vi "e.gate ReadeStateInfo.vi"(0 "Configuration  in":T1, 5 "error in (no error)":errorcluster) -> (14 "Configuration out":T1, 15 "data string":string, 16 "General States":string, 17 "Run States":string, 18 "Error States":string, 19 "error out":errorcluster)   [LabVIEW 2016]
uses:
  e.gate Configuration.ctl
  e.gate Channel Data.ctl
  e.gate Data Type.ctl
  e.gate Protocol Type.ctl
  e.gate Module  Data.ctl
  e.gateHSP_DLLhandle.ctl
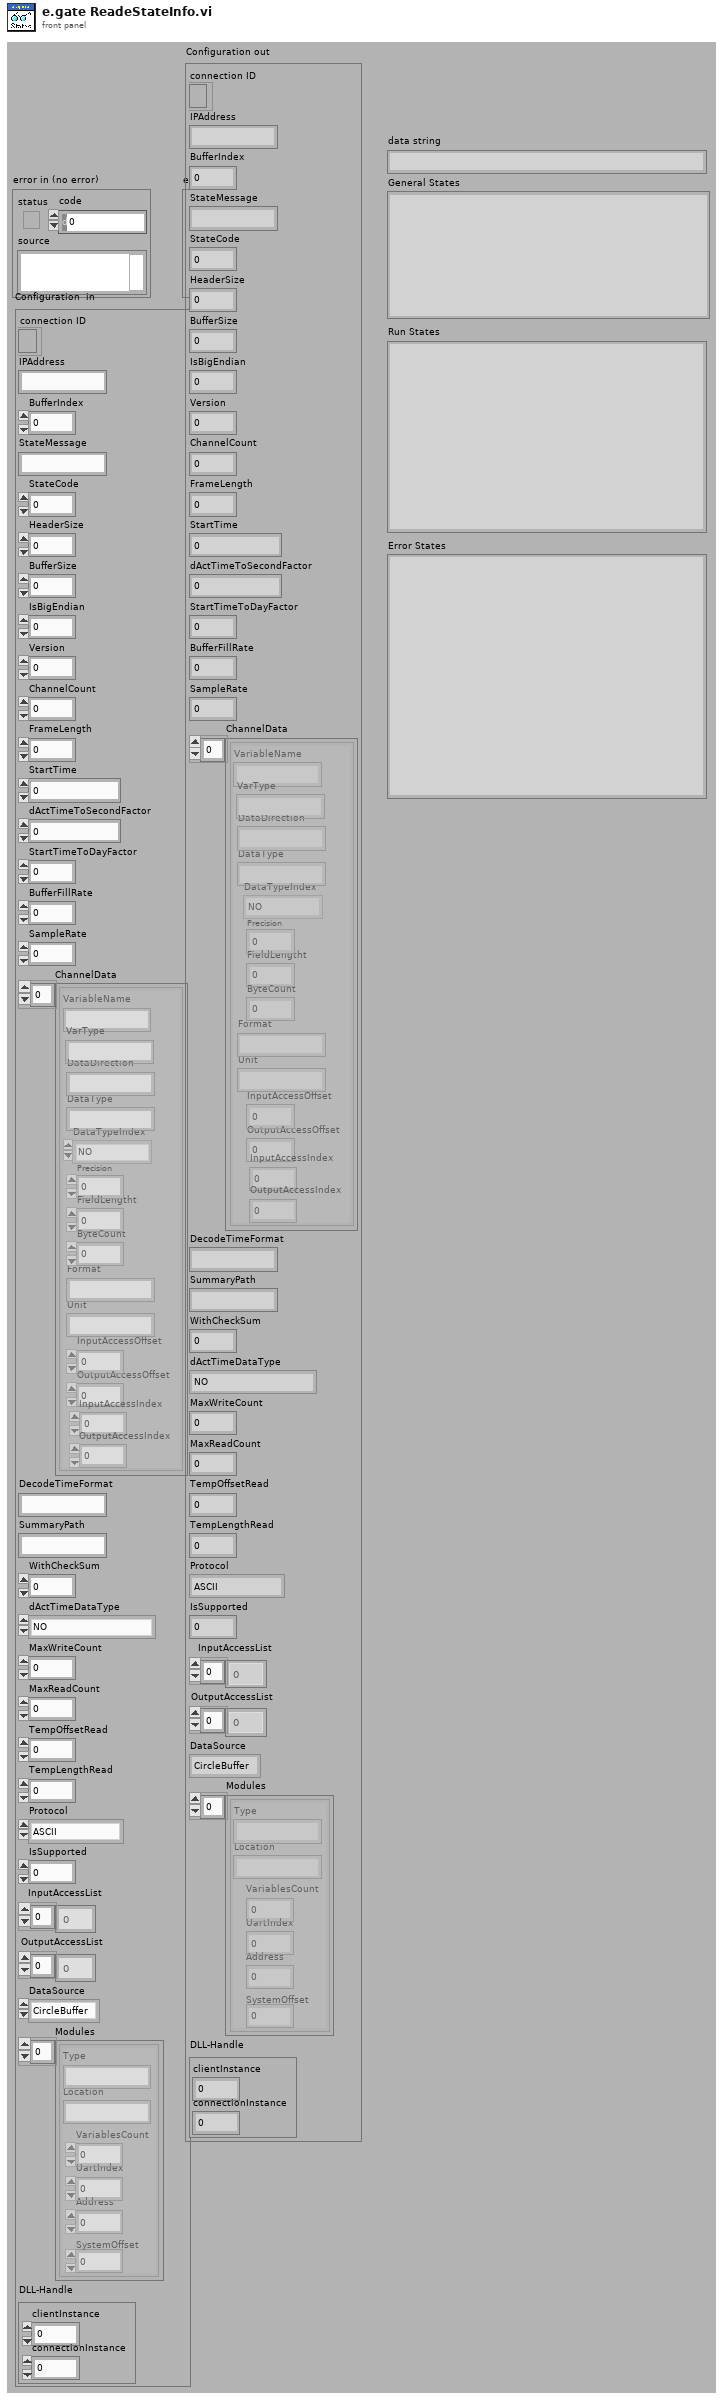
[diagram p1: front panel]
types:
  T1 = typedef "e.gate Configuration.ctl" = cluster{"connection ID":refnum<k5>, "IPAddress":string, "BufferIndex":i32, "StateMessage":string, "StateCode":i8, "HeaderSize":i32, "BufferSize":i32, "IsBigEndian":i32, "Version":i32, "ChannelCount":i32, "FrameLength":i32, "StartTime":dbl, "dActTimeToSecondFactor":dbl, "StartTimeToDayFactor":dbl, "BufferFillRate":dbl, "SampleRate":dbl, "ChannelData":T2[], "DecodeTimeFormat":string, "SummaryPath":string, "WithCheckSum":i32, "dActTimeDataType":T3, "MaxWriteCount":i32, "MaxReadCount":i32, "TempOffsetRead":i32, "TempLengthRead":i32, "Protocol":T4, "IsSupported":i32, "InputAccessList":i32[], "OutputAccessList":i32[], "DataSource":enum16{"CircleBuffer", "test.con Logger", "test.con Archive"}, "Modules":T5[], "DLL-Handle":T6}
  T2 = typedef "e.gate Channel Data.ctl" = cluster{"VariableName":string, "DataDirection":string, "DataType":string, "DataTypeIndex":T3, "Precision":i16, "FieldLengtht":i16, "ByteCount":i32, "Format":string, "Unit":string, "InputAccessOffset":i32, "OutputAccessOffset":i16, "InputAccessIndex":i16, "OutputAccessIndex":i16, "VarType":string}
  T3 = typedef "e.gate Data Type.ctl" = enum16{"NO", "BOOL", "SINT8", "USINT8", "SINT16", "USINT16", "SINT32", "USINT32", "FLOAT", "SET8", "SET16", "SET32", "DOUBLE", "SINT64", "USINT64", "SET64"}
  T4 = typedef "e.gate Protocol Type.ctl" = enum16{"ASCII", "HighspeedPort Online", "HighspeedPort Buffer", "eGateHighspeedPortDLL "}
  T5 = typedef "e.gate Module  Data.ctl" = cluster{"Type":string, "Location":string, "VariablesCount":i16, "UartIndex":i16, "Address":i16, "SystemOffset":i16}
  T6 = typedef "e.gateHSP_DLLhandle.ctl" = cluster{"clientInstance":i32, "connectionInstance":i32}
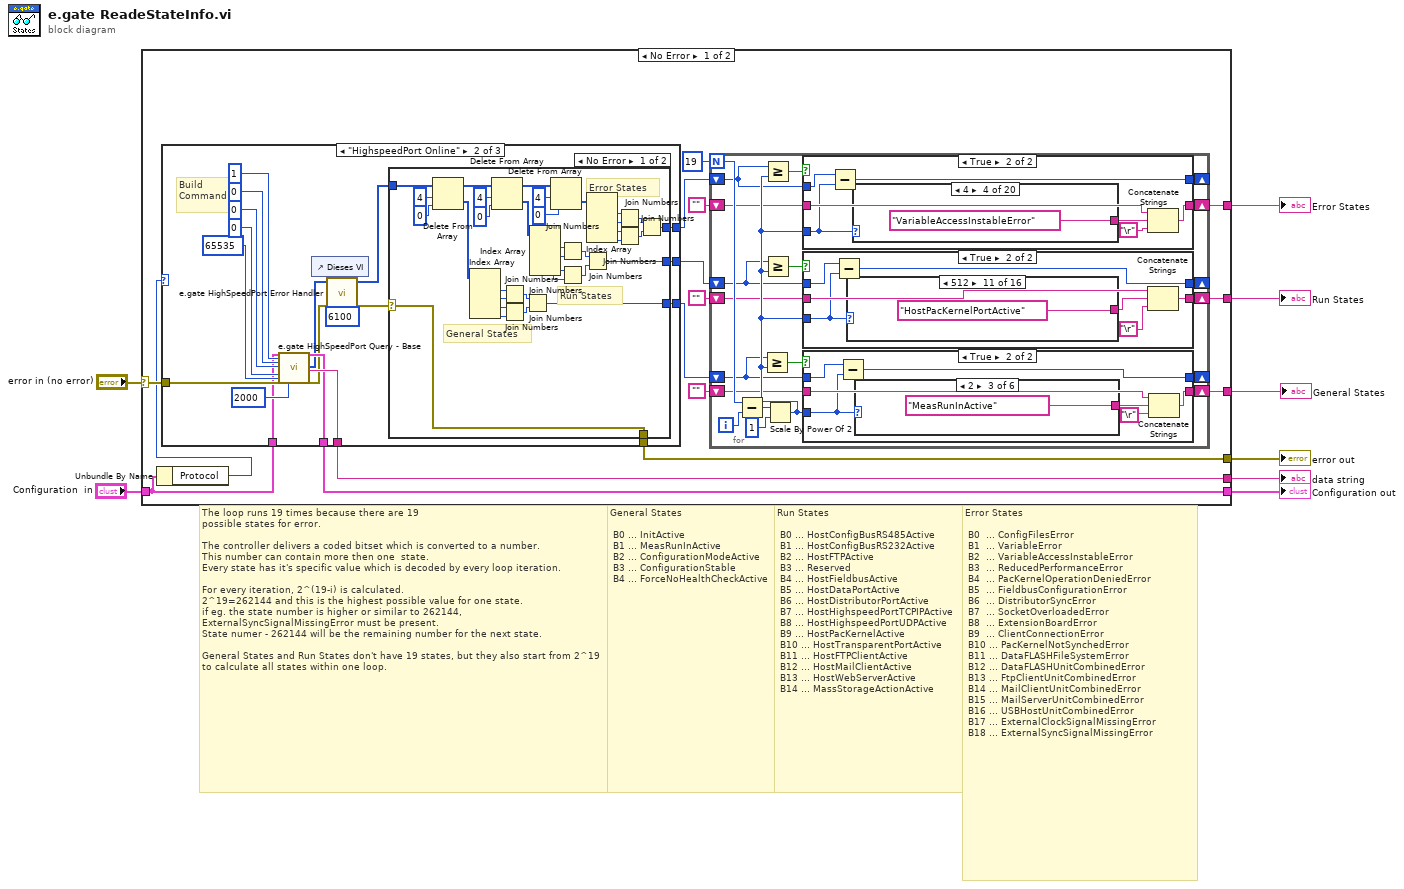
[diagram p0: block diagram]
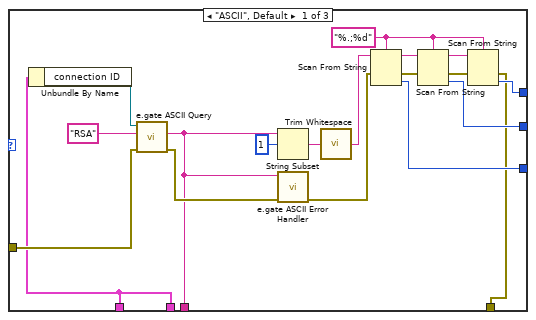
[diagram p2: hidden frame]
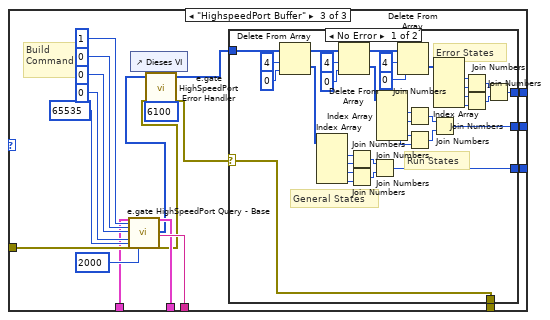
[diagram p4: hidden frame]
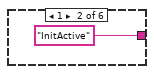
[diagram p8: hidden frame]
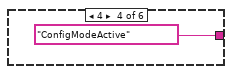
[diagram p9: hidden frame]
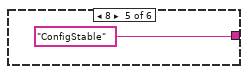
[diagram p10: hidden frame]
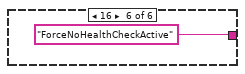
[diagram p11: hidden frame]
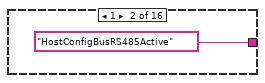
[diagram p14: hidden frame]
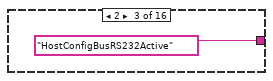
[diagram p15: hidden frame]
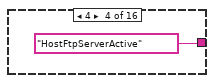
[diagram p16: hidden frame]
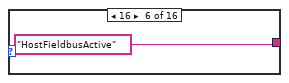
[diagram p18: hidden frame]
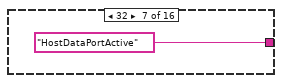
[diagram p19: hidden frame]
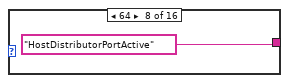
[diagram p20: hidden frame]
diagram:
  # "Error States\n\n B0\t ... ConfigFilesError \n\tB1\t ... VariableError\n\tB2\t ... VariableAccessInstableError\n\tB3\t ... ReducedPerformanceError\n B4\t ... PacKernelOperationDeniedError\n\tB5  ... FieldbusConfigurationError\n\tB6\t ... DistributorSyncError\n B7\t ... SocketOverloadedError\n\tB8\t ... ExtensionBoardError\n\tB9\t ... ClientConnectionError\n\tB10 ... PacKernelNotSynchedError\n\tB11 ... DataFLASHFileSystemError\n B12 ... DataFLASHUnitCombinedError\n\tB13 ... FtpClientUnitCombinedError\n\tB14 ... MailClientUnitCombinedError \n\tB15 ... MailServerUnitCombinedError\n\tB16 ... USBHostUnitCombinedError\n\tB17 ... ExternalClockSignalMissingError\n\tB18 ... ExternalSyncSignalMissingError"
  # "Run States\n\n\tB0 ... HostConfigBusRS485Active \n\tB1 ... HostConfigBusRS232Active \n\tB2 ... HostFTPActive \n\tB3 ... Reserved \n\tB4 ... HostFieldbusActive \n\tB5 ... HostDataPortActive\n\tB6 ... HostDistributorPortActive\n\tB7 ... HostHighspeedPortTCPIPActive\n\tB8 ... HostHighspeedPortUDPActive\n B9 ... HostPacKernelActive\n B10 ... HostTransparentPortActive\n B11 ... HostFTPClientActive\n B12 ... HostMailClientActive\n B13 ... HostWebServerActive\n B14 ... MassStorageActionActive"
  # "General States\n\n B0 ... InitActive \n\tB1 ... MeasRunInActive \n\tB2 ... ConfigurationModeActive \n\tB3 ... ConfigurationStable\n\tB4 ... ForceNoHealthCheckActive"
  # "The loop runs 19 times because there are 19\npossible states for error.\n\nThe controller delivers a coded bitset which is converted to a number.\nThis number can contain more then one  state.\nEvery state has it's specific value which is decoded by every loop iteration.\n\nFor every iteration, 2^(19-i) is calculated.\n2^19=262144 and this is the highest possible value for one state.\nif eg. the state number is higher or similar to 262144, ExternalSyncSignalMissingError must be present.\nState numer - 262144 will be the remaining number for the next state.\n\nGeneral States and Run States don't have 19 states, but they also start from 2^19 to calculate all states within one loop."
  n1 = case shown="No Error" "error in (no error)" {
    selector: "error in (no error)" -> [w24 w239]
    tunnel: [w9 w239] -> w8
    tunnel: "Configuration  in" -> [w11 w240]
    tunnel: [w10 w240] -> w5
    tunnel: [w20 _] -> w4
    tunnel: [w23 _] -> w1
    tunnel: [w22 _] -> w2
    tunnel: [w21 _] -> w3
    frame No Error {
      n2 = Unbundle By Name(w11) -> ("Protocol"=w12:T4)
      n3 = case shown="\"HighspeedPort Online\"" w12 {
        tunnel: w24 -> [w43 w63 w118]
        tunnel: [w39 w56 w111] -> w20
        tunnel: [w29 w55 w110] -> w19
        tunnel: [w30 w54 w109] -> w18
        tunnel: [w28 w53 w108] -> w17
        tunnel: w11 -> [w26 w52 w107]
        tunnel: [w26 w51 w106] -> w10
        tunnel: [w25 w44 w99] -> w9
        frame "ASCII", Default {
          w35 = "%.;%d" ("format string")
          n4 = Unbundle By Name(w26) -> ("connection ID"=w27:refnum<k5>)
          n5 = call "e.gate ASCII Query.vi"("error in (no error)"=w43, "Command"="RSA", "connection ID In"=w27) -> ("error out"=w41:errorcluster, "Response"=w39:string)  [unwired: 7 out]
          n6 = String Subset(string=w39, offset (0)=1) -> (substring=w38:string)  [unwired: 1 out]
          n7 = call "e.gate ASCII Error Handler.vi"("error in (no error)"=w41, "String"=w39) -> ("error out"=w37:errorcluster)  [unwired: 9 out]
          n8 = call <vilib>:"Trim Whitespace.vi"("string"=w38) -> ("trimmed string"=w36:string)  [unwired: 1 in]
          n9 = Scan From String(format string=w35, input string=w36, error in=w37) -> (remaining string=w34:string, error out=w32:errorcluster, output 1=w29:i32)  [unwired: 1 in, 2 out]
          n10 = Scan From String(format string=w35, input string=w34, error in=w32) -> (remaining string=w33:string, error out=w31:errorcluster, output 1=w30:i32)  [unwired: 1 in, 2 out]
          n11 = Scan From String(format string=w35, input string=w33, error in=w31) -> (error out=w25:errorcluster, output 1=w28:i32)  [unwired: 1 in, 3 out]
        }
        frame "HighspeedPort Online" {
          # "Build\nCommand"
          n12 = call "e.gate HighSpeedPort Query - Base.vi"("e.gate Configuration in"=w52, "Command"=1, "OffsetWrite"=0, "LengthWrite"=0 ("OffsetWrite"), "OffsetRead"=0, "LengthRead"=65535, "error in (no error)"=w63, "Timeout (1000)"=2000) -> ("e.gate Configuration out"=w51:T1, "Data (out binary)"=w48:u8[], "data out (string)"=w56:string, "error out"=w47:errorcluster)  [unwired: 2 in, 14 out]
          n13 = control-ref of="Dieses VI"() -> (w50:refnum<vi>)
          n14 = call "e.gate HighSpeedPort Error Handler.vi"("error code start index"=6100, "VI reference"=w50, "error in (no error)"=w47, "binary data in"=w48) -> ("error out"=w45:errorcluster, "binary out"=w46:u8[])  [unwired: 6 out]
          n15 = case shown="No Error" w45 {
            selector: w45 -> [w64 w98]
            tunnel: [w97 _] -> w55
            tunnel: [w96 _] -> w54
            tunnel: [w95 _] -> w53
            tunnel: w46 -> [w65 _]
            tunnel: [w64 w98] -> w44
            frame No Error {
              # "General States"
              # "Run States"
              # "Error States"
              n16 = Delete From Array(array=w65, length=4 ("Länge"), index=0 ("Index")) -> (deleted portion=w68:u8[], array with subset deleted=w92:u8[])
              n17 = Index Array(array=w68) -> (element #1=w91:u8, element #2=w90:u8, element #3=w84:u8, element #4=w83:u8)  [unwired: 4 in]
              n18 = Delete From Array(array=w92, length=4 ("Länge"), index=0 ("Index")) -> (deleted portion=w67:u8[], array with subset deleted=w87:u8[])
              n19 = Join Numbers(hi=w91, lo=w90) -> ((hi.lo)=w76:u16)
              n20 = Join Numbers(hi=w84, lo=w83) -> ((hi.lo)=w75:u16)
              n21 = Join Numbers(hi=w76, lo=w75) -> ((hi.lo)=w97:u32)
              n22 = Index Array(array=w67) -> (element #1=w82:u8, element #2=w81:u8, element #3=w80:u8, element #4=w70:u8)  [unwired: 4 in]
              n23 = Delete From Array(array=w87, length=4 ("Länge"), index=0 ("Index")) -> (deleted portion=w66:u8[])  [unwired: 1 out]
              n24 = Join Numbers(hi=w82, lo=w81) -> ((hi.lo)=w74:u16)
              n25 = Join Numbers(hi=w80, lo=w70) -> ((hi.lo)=w73:u16)
              n26 = Join Numbers(hi=w74, lo=w73) -> ((hi.lo)=w96:u32)
              n27 = Index Array(array=w66) -> (element #1=w79:u8, element #2=w78:u8, element #3=w77:u8, element #4=w69:u8)  [unwired: 4 in]
              n28 = Join Numbers(hi=w79, lo=w78) -> ((hi.lo)=w72:u16)
              n29 = Join Numbers(hi=w77, lo=w69) -> ((hi.lo)=w71:u16)
              n30 = Join Numbers(hi=w72, lo=w71) -> ((hi.lo)=w95:u32)
            }
            frame Error {
            }
          }
        }
        frame "HighspeedPort Buffer" {
          # "Build\nCommand"
          n31 = call "e.gate HighSpeedPort Query - Base.vi"("e.gate Configuration in"=w107, "Command"=1, "OffsetWrite"=0, "LengthWrite"=0 ("OffsetWrite"), "OffsetRead"=0, "LengthRead"=65535, "error in (no error)"=w118, "Timeout (1000)"=2000) -> ("e.gate Configuration out"=w106:T1, "Data (out binary)"=w103:u8[], "data out (string)"=w111:string, "error out"=w102:errorcluster)  [unwired: 2 in, 14 out]
          n32 = control-ref of="Dieses VI"() -> (w104:refnum<vi>)
          n33 = call "e.gate HighSpeedPort Error Handler.vi"("error code start index"=6100, "VI reference"=w104, "error in (no error)"=w102, "binary data in"=w103) -> ("error out"=w100:errorcluster, "binary out"=w101:u8[])  [unwired: 6 out]
          n34 = case shown="No Error" w100 {
            selector: w100 -> [w119 w153]
            tunnel: [w152 _] -> w110
            tunnel: [w151 _] -> w109
            tunnel: [w150 _] -> w108
            tunnel: w101 -> [w120 _]
            tunnel: [w119 w153] -> w99
            frame No Error {
              # "General States"
              # "Run States"
              # "Error States"
              n35 = Delete From Array(array=w120, length=4 ("Länge"), index=0 ("Index")) -> (deleted portion=w123:u8[], array with subset deleted=w147:u8[])
              n36 = Index Array(array=w123) -> (element #1=w146:u8, element #2=w145:u8, element #3=w139:u8, element #4=w138:u8)  [unwired: 4 in]
              n37 = Delete From Array(array=w147, length=4 ("Länge"), index=0 ("Index")) -> (deleted portion=w122:u8[], array with subset deleted=w142:u8[])
              n38 = Join Numbers(hi=w146, lo=w145) -> ((hi.lo)=w131:u16)
              n39 = Join Numbers(hi=w139, lo=w138) -> ((hi.lo)=w130:u16)
              n40 = Join Numbers(hi=w131, lo=w130) -> ((hi.lo)=w152:u32)
              n41 = Index Array(array=w122) -> (element #1=w137:u8, element #2=w136:u8, element #3=w135:u8, element #4=w125:u8)  [unwired: 4 in]
              n42 = Delete From Array(array=w142, length=4 ("Länge"), index=0 ("Index")) -> (deleted portion=w121:u8[])  [unwired: 1 out]
              n43 = Join Numbers(hi=w137, lo=w136) -> ((hi.lo)=w129:u16)
              n44 = Join Numbers(hi=w135, lo=w125) -> ((hi.lo)=w128:u16)
              n45 = Join Numbers(hi=w129, lo=w128) -> ((hi.lo)=w151:u32)
              n46 = Index Array(array=w121) -> (element #1=w134:u8, element #2=w133:u8, element #3=w132:u8, element #4=w124:u8)  [unwired: 4 in]
              n47 = Join Numbers(hi=w134, lo=w133) -> ((hi.lo)=w127:u16)
              n48 = Join Numbers(hi=w132, lo=w124) -> ((hi.lo)=w126:u16)
              n49 = Join Numbers(hi=w127, lo=w126) -> ((hi.lo)=w150:u32)
            }
            frame Error {
            }
          }
        }
      }
      n50 = for {
        N: 19 -> [w170]
        shift-right: [w160] -> w23
        shift-left: "" -> [w161]
        shift-right: [w162] -> w22
        shift-left: "" -> [w163]
        shift-right: [w164] -> w21
        shift-left: "" -> [w165]
        shift-right: [w154] -> _
        shift-left: w18 -> [w157]
        shift-right: [w158] -> _
        shift-left: w17 -> [w159]
        shift-right: [w155] -> _
        shift-left: w19 -> [w156]
        i -> [w171]
        n51 = Subtract(x=w170, y=w171) -> (x-y=w172:i32)
        n52 = Scale By Power Of 2(n=w172, x=1 ("n")) -> (x*2^n=w166:i32)
        n53 = Greater Or Equal?(x=w156, y=w166) -> (x >= y?=w167:bool)
        n54 = Greater Or Equal?(x=w159, y=w166) -> (x >= y?=w169:bool)
        n55 = Greater Or Equal?(x=w157, y=w166) -> (x >= y?=w168:bool)
        n56 = case shown="True" w169 {
          tunnel: w166 -> [_ w214]
          tunnel: w161 -> [w212 w218]
          tunnel: [w212 w217] -> w160
          tunnel: w159 -> [w211 w215]
          tunnel: [w211 w213] -> w158
          frame False {
          }
          frame True {
            n57 = Subtract(x=w215, y=w214) -> (x-y=w213:u32)
            n58 = case shown="4" w214 {
              tunnel: [_ "ConfigFilesError" "VariableError" "VariableAccessInstableError" "ReducedPerformanceError" "PacKernelOperationDeniedError" "FieldBusConfigurationError" "DirtributorSyncError" "SocketOverloadError" "ExtensionBoardError" "ClientConnectionError" "PacKernelNotSynchedError" "DataFLASHFileSystemError" "DataFLASHUnitCombinedError" "FTPClientUnitCombinedError" "MailClientUnitCombinedError" "MailServerUnitCombinedError" "USBHostUnitCombinedError" "ExternalClockSignalMissingError" "ExternalSyncSignalMissingError"] -> w216
              frame 0, Default {
              }
              frame 1 {
              }
              frame 2 {
              }
              frame 4 {
              }
              frame 8 {
              }
              frame 16 {
              }
              frame 32 {
              }
              frame 64 {
              }
              frame 128 {
              }
              frame 256 {
              }
              frame 512 {
              }
              frame 1024 {
              }
              frame 2048 {
              }
              frame 4096 {
              }
              frame 8192 {
              }
              frame 16384 {
              }
              frame 32768 {
              }
              frame 65536 {
              }
              frame 131072 {
              }
              frame 262144 {
              }
            }
            n59 = Concatenate Strings(w218, w216, "\r") -> (w217:string)
          }
        }
        n60 = case shown="True" w168 {
          tunnel: w166 -> [_ w191]
          tunnel: w163 -> [w189 w196]
          tunnel: [w189 w195] -> w162
          tunnel: w157 -> [w188 w192]
          tunnel: [w188 w190] -> w154
          frame False {
          }
          frame True {
            n61 = Subtract(x=w192, y=w191) -> (x-y=w190:u32)
            n62 = case shown="512" w191 {
              tunnel: [_ "HostConfigBusRS485Active" "HostConfigBusRS232Active" "HostFtpServerActive" _ "HostFieldbusActive" "HostDataPortActive" "HostDistributorPortActive" "HostHighspeedPortTCPIPActive" "HostHighSpeedPortUDPActive" "HostPacKernelPortActive" "HostTransparentPortActive" "HostFTPClientActive" "HostMailClientActive" "HostWebServerActive" "MassStorageActionActive"] -> w193
              frame 0, Default {
              }
              frame 1 {
              }
              frame 2 {
              }
              frame 4 {
              }
              frame 8 {
              }
              frame 16 {
              }
              frame 32 {
              }
              frame 64 {
              }
              frame 128 {
              }
              frame 256 {
              }
              frame 512 {
              }
              frame 1024 {
              }
              frame 2048 {
              }
              frame 4096 {
              }
              frame 8192 {
              }
              frame 16384 {
              }
            }
            n63 = Concatenate Strings(w196, w193, "\r") -> (w195:string)
          }
        }
        n64 = case shown="True" w167 {
          tunnel: w166 -> [_ w177]
          tunnel: w165 -> [w175 w181]
          tunnel: [w175 w180] -> w164
          tunnel: w156 -> [w174 w178]
          tunnel: [w174 w176] -> w155
          frame False {
          }
          frame True {
            n65 = Subtract(x=w178, y=w177) -> (x-y=w176:u32)
            n66 = case shown="2" w177 {
              tunnel: [_ "InitActive" "MeasRunInActive" "ConfigModeActive" "ConfigStable" "ForceNoHealthCheckActive"] -> w179
              frame 0, Default {
              }
              frame 1 {
              }
              frame 2 {
              }
              frame 4 {
              }
              frame 8 {
              }
              frame 16 {
              }
            }
            n67 = Concatenate Strings(w181, w179, "\r") -> (w180:string)
          }
        }
      }
    }
    frame Error {
    }
  }
  "error out" <- w8
  "Configuration out" <- w5
  "data string" <- w4
  "General States" <- w3
  "Run States" <- w2
  "Error States" <- w1
